vi "Remove RS485 Address.vi"(4 "error in":errorcluster, 6 "Command (input)":string, 7 "VISA resource name in":refnum<visa-resource-name>) -> (0 "error out":errorcluster, 2 "Command (output)":string, 3 "VISA resource name out":refnum<visa-resource-name>)   [LabVIEW 2015, in "JULABO DeviceDriver.lvlib"]
uses:
  JULABO DeviceDriver.lvlib
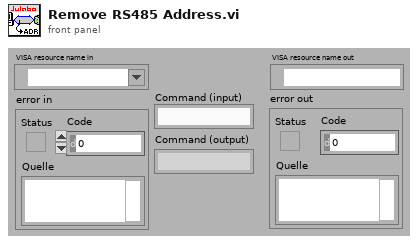
[diagram p1: front panel]
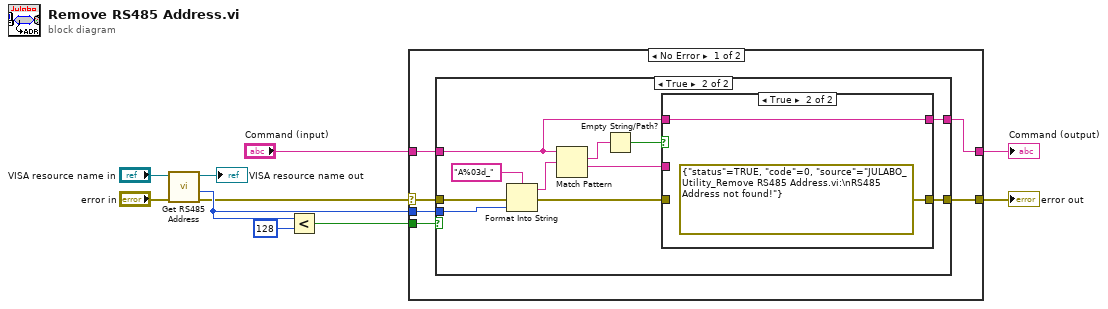
[diagram p0: block diagram]
diagram:
  n1 = call "Get RS485 Address.vi"("error in"="error in", "VISA resource name in"="VISA resource name in") -> ("Fehler (Ausgang)"=w1:errorcluster, "RS485-Address"=w2:u8, "VISA resource name out"=→"VISA resource name out":refnum<visa-resource-name>)  [unwired: 3 in]
  n2 = Less?(x=w2, y=u32 128) -> (x < y?=w9:bool)
  n3 = case shown="No Error" w1 {
    selector: w1 -> [w11 w35]
    tunnel: w9 -> [w16 _]
    tunnel: [w15 w34] -> w8
    tunnel: "Command (input)" -> [w14 w34]
    tunnel: [w13 w35] -> w6
    tunnel: w2 -> [w12 _]
    frame No Error {
      n4 = case shown="True" w16 {
        tunnel: [w18 w24] -> w15
        tunnel: w14 -> [w18 w20]
        tunnel: w11 -> [w17 w29]
        tunnel: w12 -> [_ w28]
        tunnel: [w17 w22] -> w13
        frame False {
        }
        frame True {
          n5 = Format Into String(format string="A%03d_" ("Format-String"), error in=w29, w28) -> (resulting string=w26:string, error out=w21:errorcluster)  [unwired: 1 in]
          n6 = Match Pattern(string=w20, regular expression=w26) -> (match substring=w23:string, after substring=w19:string)  [unwired: 1 in, 2 out]
          n7 = Empty String/Path?(string/path=w23) -> (empty?=w25:bool)
          n8 = case shown="True" w25 {
            tunnel: [w31 w33] -> w24
            tunnel: w19 -> [w31 _]
            tunnel: [w30 errorcluster {"status"=TRUE, "code"=0, "source"="JULABO_Utility_Remove RS485 Address.vi:\nRS485 Address not found!"} ("error IO")] -> w22
            tunnel: w21 -> [w30 _]
            tunnel: w20 -> [_ w33]
            frame False {
            }
            frame True {
            }
          }
        }
      }
    }
    frame Error {
    }
  }
  "error out" <- w6
  "Command (output)" <- w8
